vi "Write Operation Selection Rule.vi"(8 "error in (no error)":errorcluster, 10 "Operation Seletion Rule":T1=enum."SPT", 11 "Scheduler in":refnum<class "Scheduler.lvclass">) -> (0 "error out":errorcluster, 3 "Scheduler out":refnum<class "Scheduler.lvclass">)   [LabVIEW 2013, in "Scheduler.lvclass"]
uses:
  Scheduler.lvclass
  Modified GT Active Scheduler/Operation Selection Rule from Subset to Schedule.ctl
  Scheduler.lvclass/Scheduler.ctl
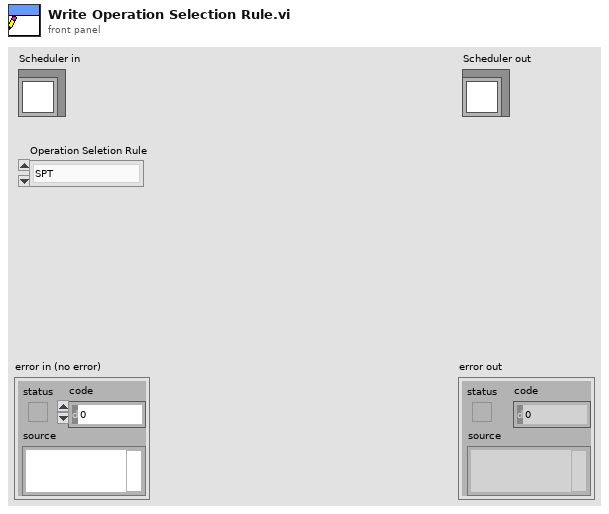
[diagram p1: front panel]
types:
  T1 = typedef "Scheduler.lvclass/Operation Selection Rule from Subset to Schedule.ctl" = enum16{"First Operation in Order", "SPT", "EDD", "MDD"}
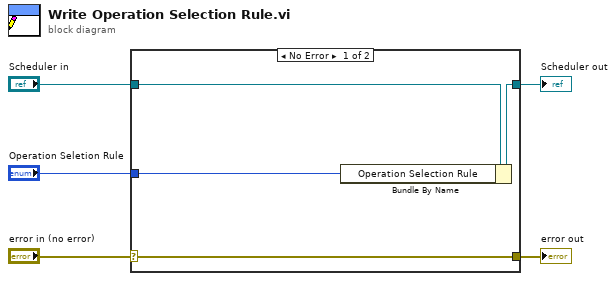
[diagram p0: block diagram]
diagram:
  n1 = case shown="No Error" "error in (no error)" {
    selector: "error in (no error)" -> [w9 w10]
    tunnel: [w9 w10] -> w4
    tunnel: [w7 w11] -> w2
    tunnel: "Scheduler in" -> [w8 w11]
    tunnel: "Operation Seletion Rule" -> [w6 _]
    frame No Error {
      n2 = Bundle By Name(cluster=w8, "Operation Selection Rule"=w6) -> (w7:refnum<class "Scheduler.lvclass">)
    }
    frame Error {
    }
  }
  "error out" <- w4
  "Scheduler out" <- w2
